vi "Write Color.vi"(4 "Symbol":T1, 6 "Color":u32(colorbox), 7 "Options":T2, 9 "Tree Tag":string, 10 "error in (no error)":errorcluster, 11 "Tree in":refnum<vi>) -> (0 "error out":errorcluster, 1 "Tree Tag (dup)":string, 3 "Tree out":refnum<vi>)   [LabVIEW 2019, in "BlueVariantView.lvlib"]
uses:
  BlueVariantView.lvlib
  API/Typedefs/Options.ctl
  Symbol.ctl
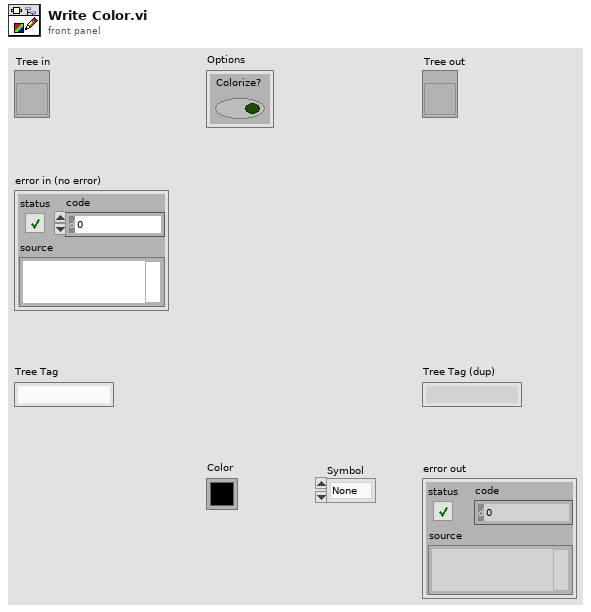
[diagram p1: front panel]
types:
  T1 = typedef "BlueVariantView.lvlib/Symbol.ctl" = enum16{"None", "Cluster-brown", "Cluster-yellow", "Cluster-black", "Cluster-pink", "Array", "Float", "Int", "Bool", "String", "Enum", "Object", "Map", "Set", "Refnum", "Variant", "Path", "Picture", "Waveform", "Timestamp", "Digital Waveform", "Fixed Point"}
  T2 = typedef "BlueVariantView.lvlib/Options.ctl" = cluster{"Colorize?":bool}
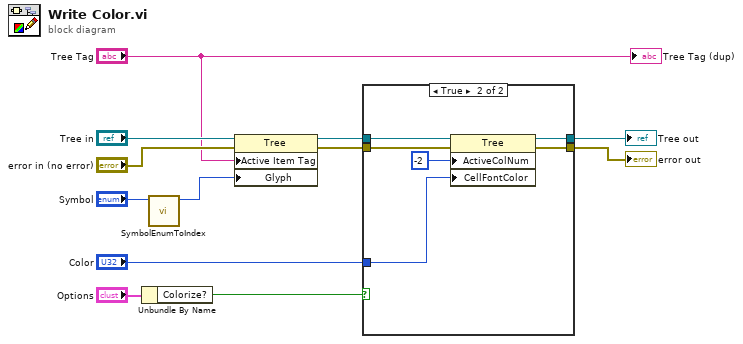
[diagram p0: block diagram]
diagram:
  n1 = Unbundle By Name("Options") -> ("Colorize?"=w11:bool)
  n2 = call "SymbolEnumToIndex.vi"("symbol enum"="Symbol") -> ("ItemSyms"=w3:i32)  [unwired: 10 in]
  n3 = property class="Tree"(reference="Tree in", error in="error in (no error)", "Active Item Tag"="Tree Tag", "Glyph"=w3) -> (reference out=w2:refnum<vi>, error out=w1:errorcluster)
  n4 = case shown="True" w11 {
    tunnel: w2 -> [w13 w20]
    tunnel: w1 -> [w14 w19]
    tunnel: "Color" -> [_ w15]
    tunnel: [w14 w17] -> w9
    tunnel: [w13 w16] -> w10
    frame False {
    }
    frame True {
      n5 = property class="Tree"(reference=w20, error in=w19, "ActiveColNum"=-2 ("Active Cell:Active Column Number"), "CellFontColor"=w15) -> (reference out=w16:refnum<vi>, error out=w17:errorcluster)
    }
  }
  "Tree out" <- w10
  "error out" <- w9
  "Tree Tag (dup)" <- "Tree Tag"
